vi "Excel_Read_String_Array.vi"(4 "Cell Range 2":string="C2", 6 "Cell Range 1":string="C2", 7 "Worksheet Number":i32=1, 8 "error in (no error)":errorcluster, 9 "Sheets Reference In":refnum<k7>) -> (0 "error out":errorcluster, 1 "Sheets Reference Out":refnum<k7>, 2 "String Array":string[][](array[string]))   [LabVIEW 2014]
doc: "This VI demonstrates the use of ActiveX to write a table into a Microsoft Excel worksheet."
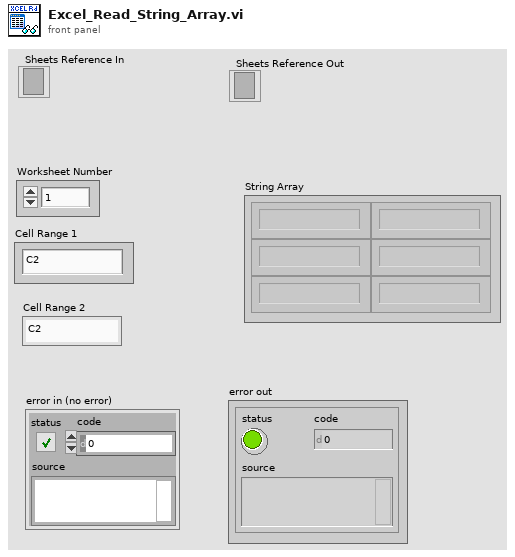
[diagram p1: front panel]
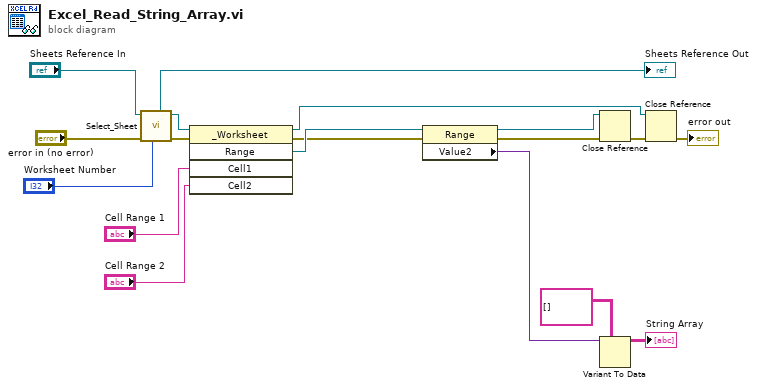
[diagram p0: block diagram]
diagram:
  n1 = call "Select_Sheet.vi"("Worksheet Number"="Worksheet Number", "error in (no error)"="error in (no error)", "Automation Refnum in"="Sheets Reference In") -> ("error out"=w5:errorcluster, "Automation Refnum out"=w7:refnum<k7>, "Sheets Refnum"=→"Sheets Reference Out":refnum<k7>)  [unwired: 6 in]
  n2 = invoke class="_Worksheet" method="Range"(reference=w7, error in=w5, "Cell1"="Cell Range 1", "Cell2"="Cell Range 2") -> (reference out=w6:refnum<k7>, error out=w11:errorcluster, "Range"=w12:refnum<k7>)  [unwired: 1 in, 2 out]
  n3 = property class="Range"(reference=w12, error in=w11) -> (reference out=w10:refnum<k7>, error out=w9:errorcluster, "Value2"=w13:variant)
  n4 = Close Reference(reference=w10, error in (no error)=w9) -> (error out=w4:errorcluster)
  n5 = Variant To Data(type=string[][] [], Variant=w13) -> (data=→"String Array":string[][])  [unwired: 1 in, 1 out]
  n6 = Close Reference(reference=w6, error in (no error)=w4) -> (error out=→"error out":errorcluster)
